vi "Client requests.vi"(8 "error in":errorcluster) -> (0 "error out":errorcluster, 1 "Good request":bool, 2 "Number of Pending Requests":i32, 3 "DesignRequest":T2, 4 "Successful Checkout":bool)   [LabVIEW 2012, in "Design Server.lvlib"]
uses:
  Design Server.lvlib
  Design Request.ctl
  Variable cluster.ctl
  user project design.ctl
  Folders.ctl
panel:
  in  "request datatype":T1
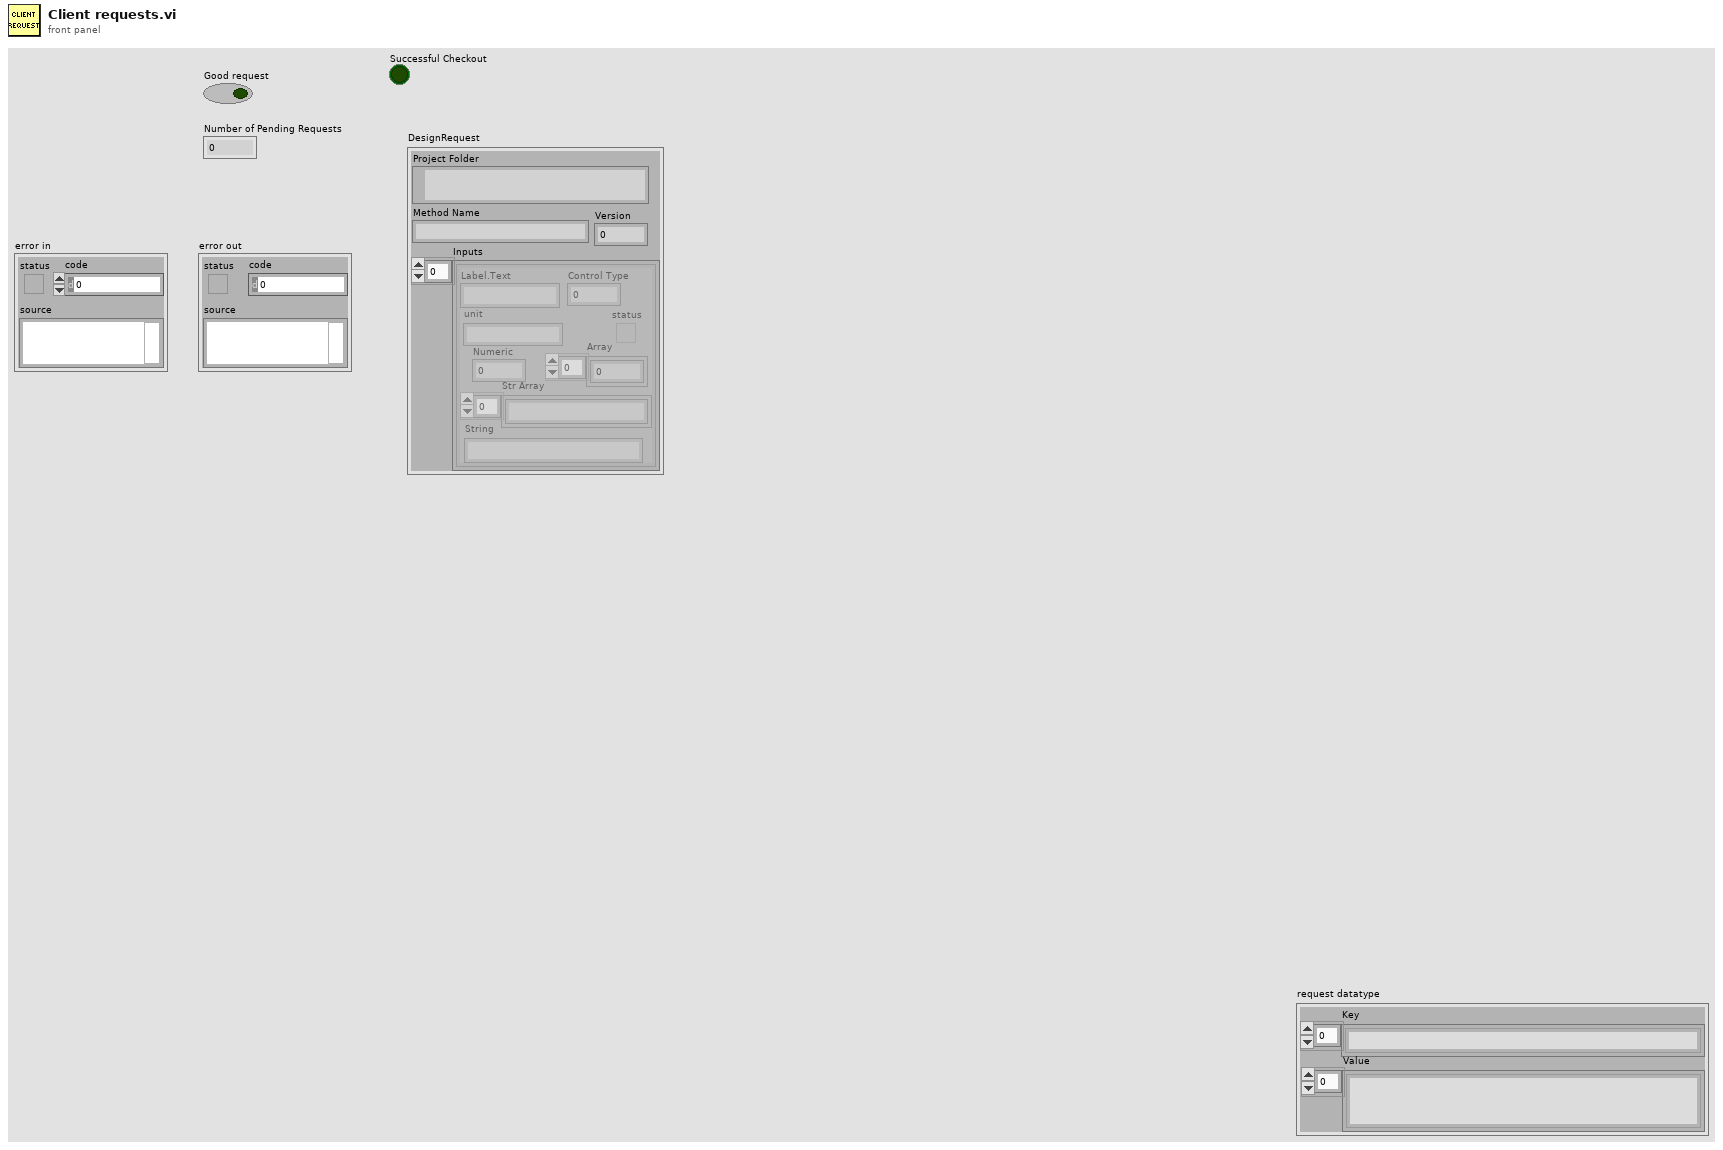
[diagram p1: front panel]
types:
  T1 = typedef "Design Server.lvlib/user project design.ctl" = cluster{"Key":string[], "Value":string[]}
  T2 = typedef "Design Server.lvlib/Design Request.ctl" = cluster{"Project Folder":path, "Method Name":string, "Inputs":T3, "Version":i32}
  T3 = typedef "Design Server.lvlib/Variable cluster.ctl" = cluster{"Label.Text":string, "Control Type":u32, "Numeric":dbl, "Array":dbl[], "status":bool, "Str Array":string[], "String":string, "unit":string}[]
  T4 = typedef "Design Server.lvlib/Folders.ctl" = enum16{"MathcadMethods", "RequestedDesigns", "CompletedDesigns", "MathcadCode", "CollabnetSVN.exe"}
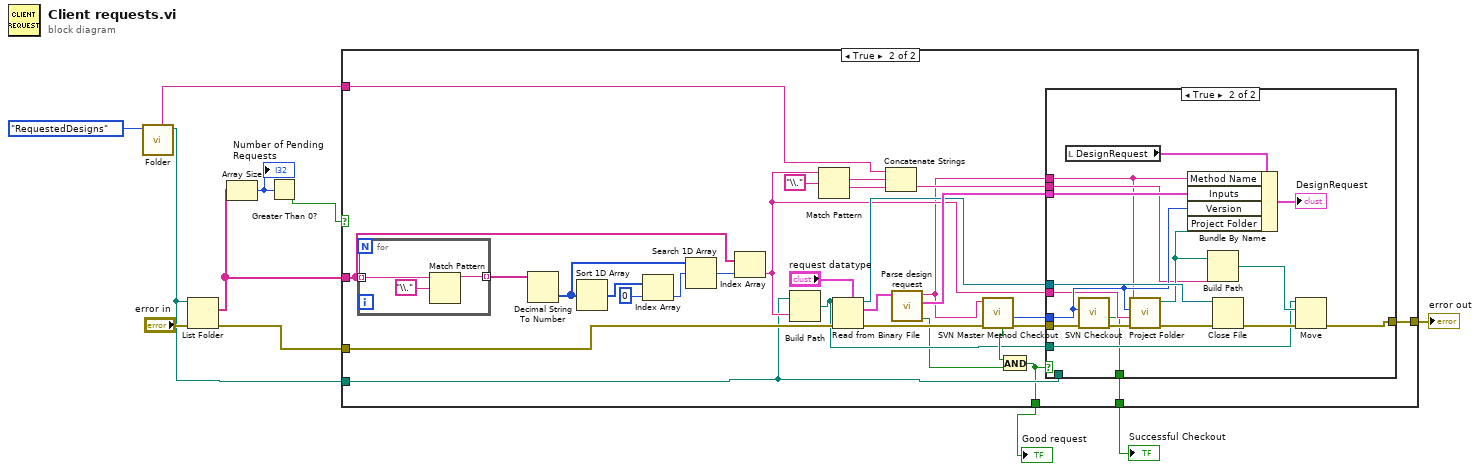
[diagram p0: block diagram]
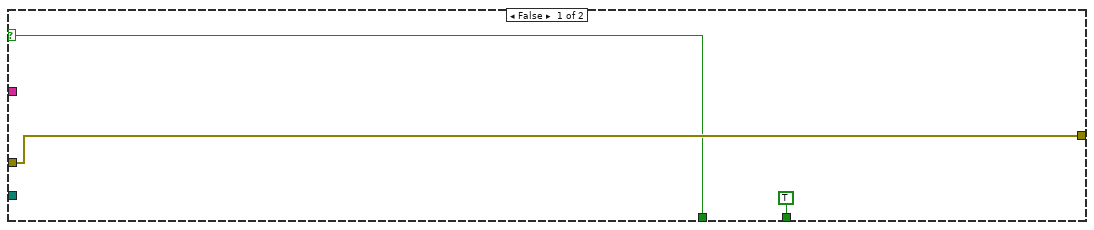
[diagram p2: hidden frame]
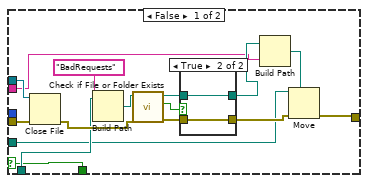
[diagram p3: hidden frame]
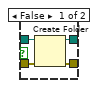
[diagram p4: hidden frame]
diagram:
  n1 = call "Folder.vi"("Folders"=Folders."RequestedDesigns") -> ("FolderPath"=w5:path, "Folder name"=w6:string)  [unwired: 8 in, 1 out]
  n2 = List Folder(path=w5, error in="error in") -> (filenames=w8:string[], error out=w7:errorcluster)  [unwired: 2 in, 2 out]
  n3 = Array Size(array=w8) -> (size(s)=w10:i32)
  "Number of Pending Requests" <- w10
  n4 = Greater Than 0?(x=w10) -> (x > 0?=w2:bool)
  n5 = case shown="True" w2 {
    selector: w2 -> [w13 _]
    tunnel: w8 -> [_ w43]
    tunnel: w7 -> [w14 w42]
    tunnel: w6 -> [_ w35]
    tunnel: w5 -> [_ w19]
    tunnel: [w14 w32] -> w4
    tunnel: [w13 w18] -> w1
    tunnel: [TRUE ("Successful Checkout") w17] -> w3
    frame False {
    }
    frame True {
      n6 = for {
        tunnel: w43 -> [w85] mode=indexing
        tunnel: [w83] -> w31 mode=indexing
        n7 = Match Pattern(string=w85, regular expression="\\.") -> (before substring=w83:string)  [unwired: 1 in, 3 out]
      }
      n8 = Decimal String To Number(string=w31) -> (number=w29:i32[])  [unwired: 2 in, 1 out]
      n9 = Sort 1D Array(array=w29) -> (sorted array=w27:i32[])
      n10 = Index Array(array=w27, index=0) -> (element=w28:i32)
      n11 = Search 1D Array(1D array=w29, element=w28) -> (index of element=w30:i32)  [unwired: 1 in]
      n12 = Index Array(array=w43, index=w30) -> (element=w33:string)
      n13 = Build Path(base path=w19, name or relative path=w33) -> (appended path=w20:path)
      n14 = Match Pattern(string=w33, regular expression="\\.") -> (match substring=w38:string, after substring=w39:string)  [unwired: 1 in, 2 out]
      n15 = Read from Binary File(5:"request datatype", 8:w42, 11:w20) -> (0:w23:errorcluster, 2:w24:T1, 3:w36:refnum<file>)  [unwired: 3 in, 1 out]
      n16 = Concatenate Strings(w35, w38, w39) -> (w37:string)
      n17 = call "Parse design request.vi"("Request"=w24) -> ("Good Method"=w16:bool, "User and project info"=w41:T3, "Method"=w15:string)  [unwired: 7 in, 1 out]
      n18 = call "SVN Master Method Checkout.vi"("error in (no error)"=w23, "Method Name"=w15) -> ("error out"=w22:errorcluster, "Method Version"=w34:i32, "Method Exists"=w21:bool)  [unwired: 4 in, 3 out]
      n19 = And(x=w21, y=w16) -> (x .and. y?=w18:bool)
      n20 = case shown="True" w18 {
        selector: w18 -> [w46 _]
        tunnel: w41 -> [_ w80]
        tunnel: w15 -> [_ w66]
        tunnel: w37 -> [_ w68]
        tunnel: w36 -> [w57 w77]
        tunnel: w20 -> [w44 w76]
        tunnel: w34 -> [_ w73]
        tunnel: w33 -> [w45 w72]
        tunnel: [w58 w70] -> w32
        tunnel: w22 -> [w59 w69]
        tunnel: w19 -> [w49 _]
        tunnel: [w46 w67] -> w17
        frame False {
          n21 = Close File(refnum=w57, error in=w59) -> (error out=w51:errorcluster)  [unwired: 1 out]
          n22 = Build Path(base path=w49, name or relative path="BadRequests") -> (appended path=w55:path)
          n23 = call <vilib>:"Check if File or Folder Exists.vi"("error in (no error)"=w51, "path"=w55) -> ("error out"=w54:errorcluster, "file or folder exists?"=w52:bool, "dup path"=w53:path)  [unwired: 7 in]
          n24 = case shown="True" w52 {
            tunnel: w54 -> [w63 w65]
            tunnel: w53 -> [w62 w64]
            tunnel: [w61 w65] -> w50
            tunnel: [w60 w64] -> w48
            frame False {
              n25 = Create Folder(path (use dialog)=w62, error in=w63) -> (created path=w60:path, error out=w61:errorcluster)  [unwired: 1 in, 1 out]
            }
            frame True {
            }
          }
          n26 = Build Path(base path=w48, name or relative path=w45) -> (appended path=w47:path)
          n27 = Move(source path=w44, error in=w50, 10:w47) -> (error out=w58:errorcluster)  [unwired: 2 in, 2 out]
        }
        frame True {
          n28 = local read "DesignRequest"() -> (w82:T2)
          n29 = call "SVN Checkout.vi"("error in (no error)"=w69, "ADT version"=w73) -> ("error out"=w75:errorcluster, "Successful Checkout"=w67:bool)  [unwired: 6 in, 2 out]
          n30 = call "Project Folder.vi"("error in (no error)"=w75, "Request File Name"=w72, "Revision"=w73, "Method"=w66) -> ("error out"=w74:errorcluster, "Completed Design path"=w71:path)  [unwired: 6 in]
          n31 = Bundle By Name(cluster=w82, "Method Name"=w66, "Inputs"=w80, "Version"=w73, "Project Folder"=w71) -> (→"DesignRequest":T2)
          n32 = Build Path(base path=w71, name or relative path=w68) -> (appended path=w78:path)
          n33 = Close File(refnum=w77, error in=w74) -> (error out=w79:errorcluster)  [unwired: 1 out]
          n34 = Move(source path=w76, error in=w79, 10:w78) -> (error out=w70:errorcluster)  [unwired: 2 in, 2 out]
        }
      }
    }
  }
  "error out" <- w4
  "Good request" <- w1
  "Successful Checkout" <- w3
